vi "test_Set-Get PCL Decimation.vi"(8 "error in (no error)":errorcluster, 11 "TestCase in":refnum<class "Instrument Addon Scripting API Custom Device Unit Tests.lvclass">) -> (0 "error out":errorcluster, 3 "TestCase out":refnum<class "Instrument Addon Scripting API Custom Device Unit Tests.lvclass">)   [LabVIEW 2019, in "Instrument Addon Scripting API Custom Device Unit Tests.lvclass"]
uses:
  Instrument Addon Scripting API Custom Device Unit Tests.lvclass
  <vilib>/addons/_JKI Toolkits/VI Tester/TestCase.llb/TestCase.lvclass
  APIs/Scripting API/Instrument Addon Scripting API.lvlib
  C:/Program Files (x86)/National Instruments/LabVIEW 2019/vi.lib/addons/_JKI Toolkits/VI Tester/TestCase.llb/TestCase.lvclass
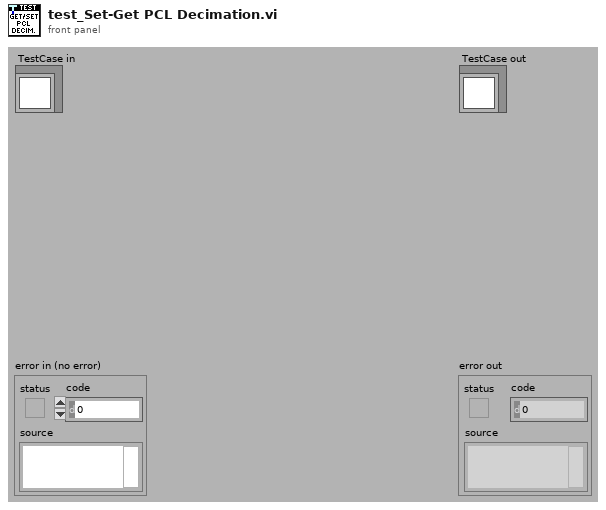
[diagram p1: front panel]
types:
  T1 = typedef "Custom Device API.lvlib/Custom Device Item Ref.ctl" = u64
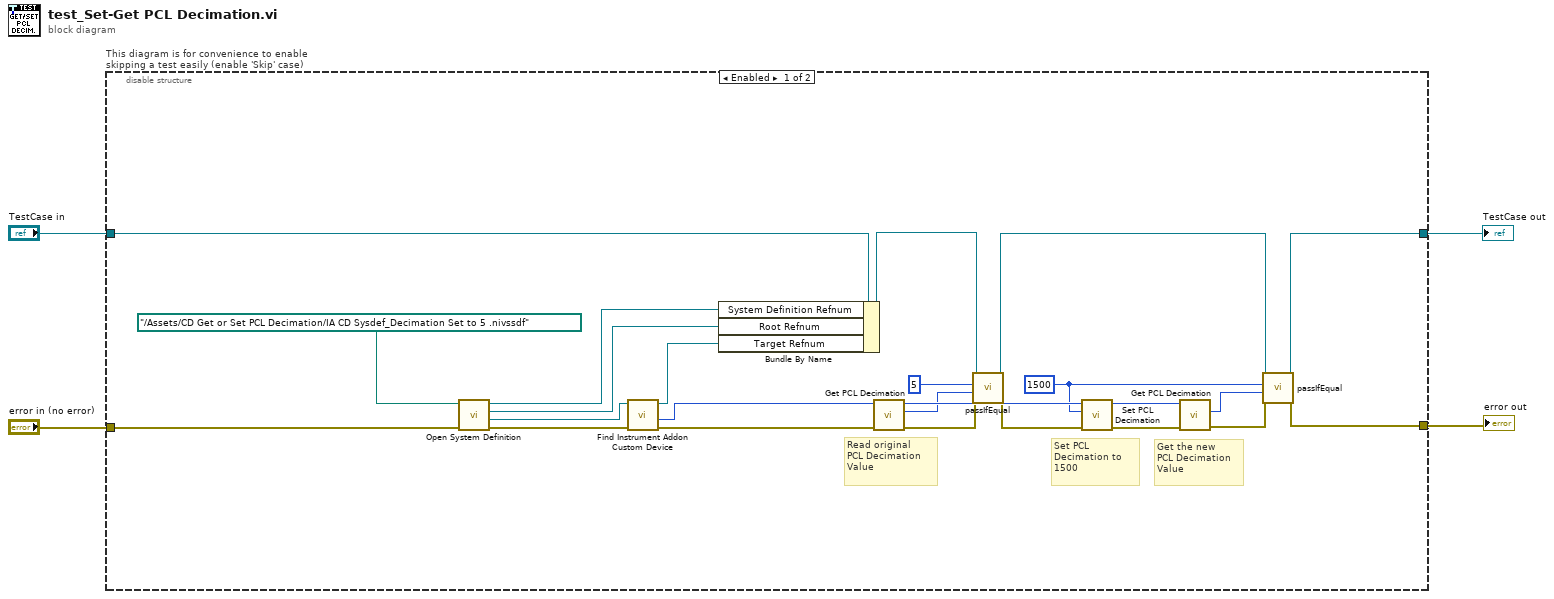
[diagram p0: block diagram]
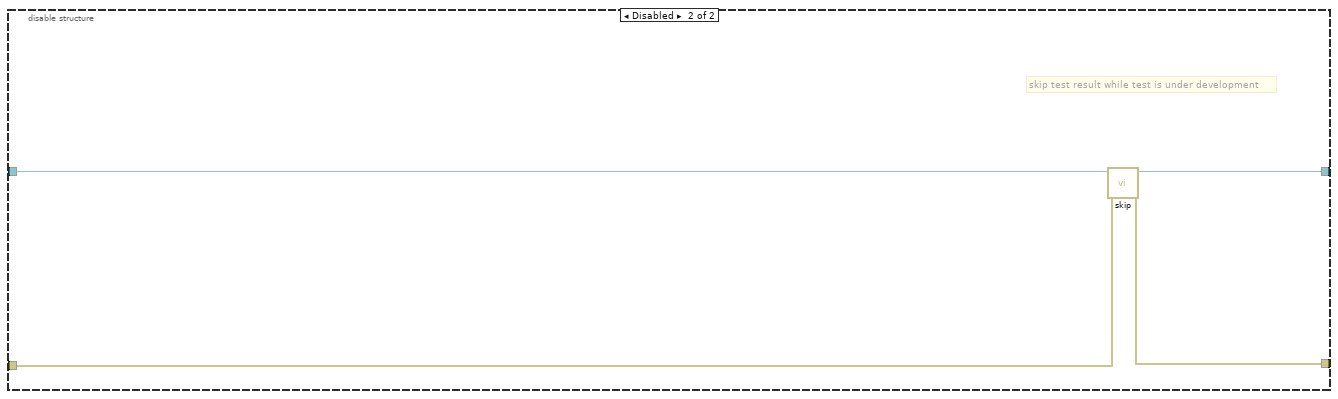
[diagram p2: hidden frame]
diagram:
  n1 = disable-structure "This diagram is for convenience to enable skipping a test easily (enable 'Skip' case)" shown="Enabled" {
    disable-tunnel: "TestCase in" -> [w9 w32]
    disable-tunnel: [w28 w30] -> w1
    disable-tunnel: [w27 w31] -> w3
    disable-tunnel: "error in (no error)" -> [w26 w29]
    frame Enabled {
      w10 = u32 1500 ("PCL Decimation")
      # "Get the new\nPCL Decimation\nValue"
      # "Set PCL Decimation to\n1500"
      # "Read original \nPCL Decimation \nValue"
      n2 = call "Open System Definition.vi"("error in (no error)"=w26, "System Definition File"=path "../Assets/CD Get or Set PCL Decimation/IA CD Sysdef_Decimation Set to 5 .nivssdf") -> ("error out"=w19:errorcluster, "Target Refnum"=w24:refnum<k24>, "Root Refnum"=w6:refnum<k24>, "System Definition Refnum"=w7:refnum<k24>)  [unwired: 6 in]
      n3 = call "Find Instrument Addon Custom Device.vi"("error in"=w19, "target in"=w24) -> ("error out"=w18:errorcluster, "NodeID"=w17:u64, "target out"=w5:refnum<k24>)  [unwired: 7 in]
      n4 = Bundle By Name(cluster=w9, "System Definition Refnum"=w7, "Root Refnum"=w6, "Target Refnum"=w5) -> (w8:refnum<class "Instrument Addon Scripting API Custom Device Unit Tests.lvclass">)
      n5 = call "Get PCL Decimation.vi"("error in (no error)"=w18, "instrument addon refnum in"=w17) -> ("error out"=w14:errorcluster, "PCL decimation"=w12:u32, "instrument addon refnum out"=w16:T1)  [unwired: 7 in]
      n6 = call-dynamic "passIfEqual.vi"("error in (no error)"=w14, "y"=w12, "x"=u32 5 ("PCL Decimation"), "TestCase in"=w8) -> ("error out"=w13:errorcluster, "TestCase out"=w15:refnum<class "Instrument Addon Scripting API Custom Device Unit Tests.lvclass">)  [unwired: 6 in]
      n7 = call "Set PCL Decimation.vi"("error in (no error)"=w13, "PCL decimation"=w10, "instrument addon refnum in"=w16) -> ("error out"=w23:errorcluster, "instrument addon refnum"=w22:T1)  [unwired: 7 in]
      n8 = call "Get PCL Decimation.vi"("error in (no error)"=w23, "instrument addon refnum in"=w22) -> ("error out"=w21:errorcluster, "PCL decimation"=w20:u32)  [unwired: 7 in, 1 out]
      n9 = call-dynamic "passIfEqual.vi"("error in (no error)"=w21, "y"=w20, "x"=w10, "TestCase in"=w15) -> ("error out"=w27:errorcluster, "TestCase out"=w28:refnum<class "Instrument Addon Scripting API Custom Device Unit Tests.lvclass">)  [unwired: 6 in]
    }
    frame Disabled {
      # "skip test result while test is under development"
      n10 = call <vilib>:"skip.vi"("error in (no error)"=w29, "TestCase in"=w32) -> ("error out"=w31:errorcluster, "TestCase out"=w30:refnum<class "Instrument Addon Scripting API Custom Device Unit Tests.lvclass">)  [unwired: 8 in]
    }
  }
  "error out" <- w3
  "TestCase out" <- w1
